vi "加速度信号处理.vi"(0 "输入信号":dbl[](graph), 1 "n":i32=2) -> (6 "滤波":dbl[](graph), 7 "重心频率FC":dbl, 8 "幅度谱":dbl[](graph), 9 "均方频率MSF":dbl, 10 "相位谱":dbl[](graph), 11 "去均值":dbl[](graph), 12 "功率谱":dbl[](graph), 13 "频率方差VF":dbl, 14 "均方根值":dbl format="%f", 15 "峰值指标":dbl format="%0.2p", 16 "峭度指标":dbl format="%0.2p", 17 "波形指标":dbl format="%0.2p", 18 "脉冲指标":dbl format="%0.2p", 19 "裕度指标":dbl format="%0.2p")   [LabVIEW 2014]
uses:
  <vilib>/Analysis/3filter.llb/Filter Passband Type.ctl
  <vilib>/Analysis/2dsp.llb/Power Spectrum (DBL).vi
  <vilib>/Analysis/3filter.llb/Butterworth Filter (DBL).vi
  <vilib>/measure/madcrms.llb/Basic Averaged DC-RMS for 1 Chan.vi
  <vilib>/Analysis/NI_AALBase.lvlib
  <vilib>/measure/NI_MAPro.lvlib
  <vilib>/Analysis/NI_AALPro.lvlib
panel:
  out "Power Spectrum":dbl[](array[numeric]) caption="功率谱"
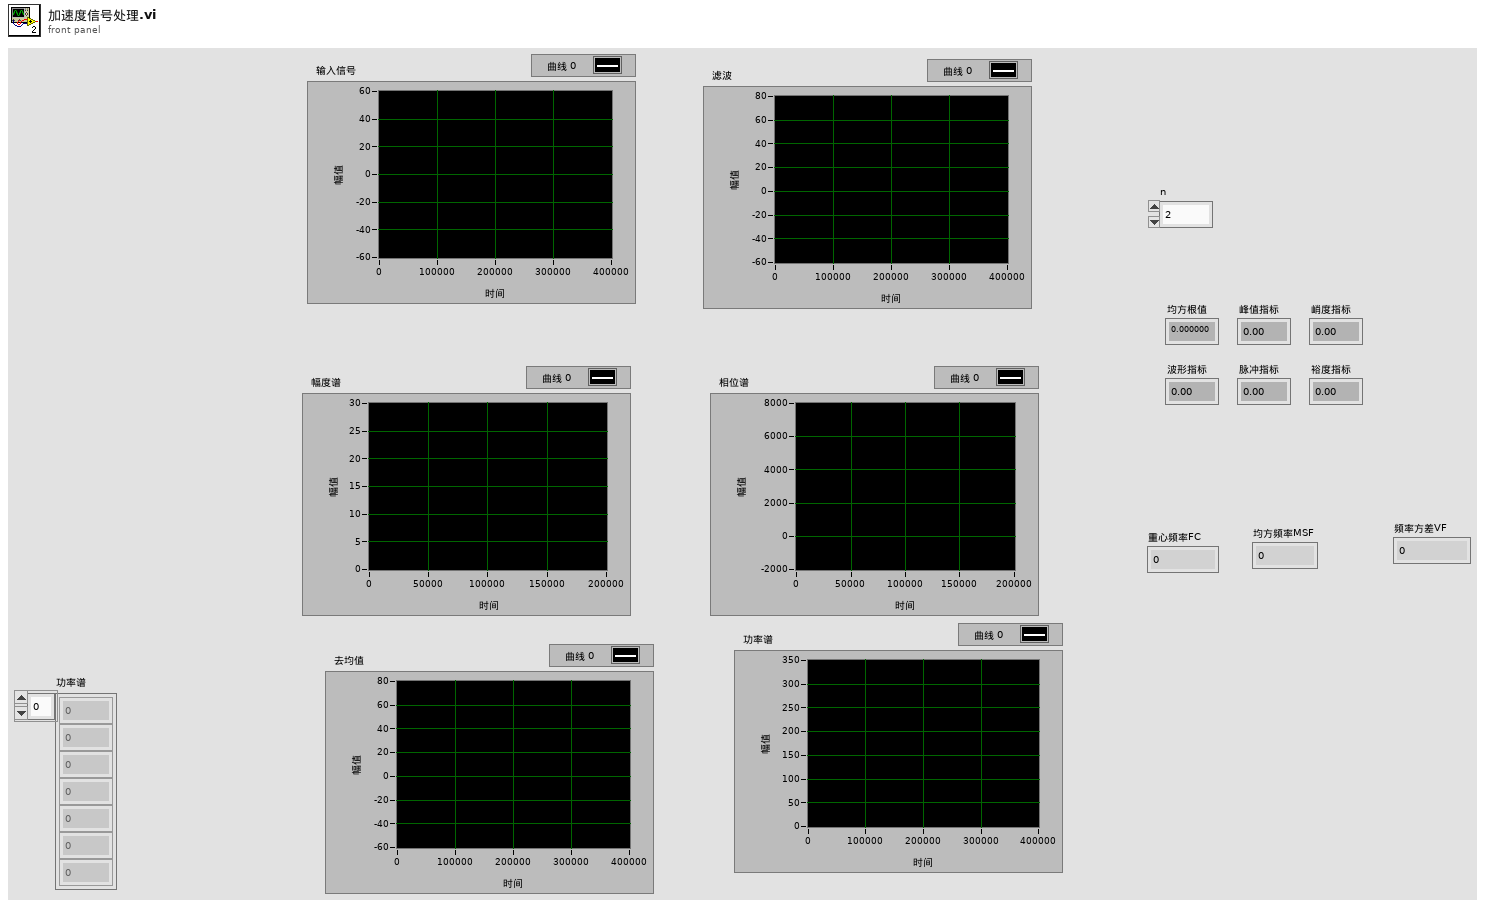
[diagram p1: front panel]
types:
  T1 = typedef "NI_AALBase.lvlib/Filter Passband Type.ctl" = enum32{"Lowpass", "Highpass", "Bandpass", "Bandstop"}
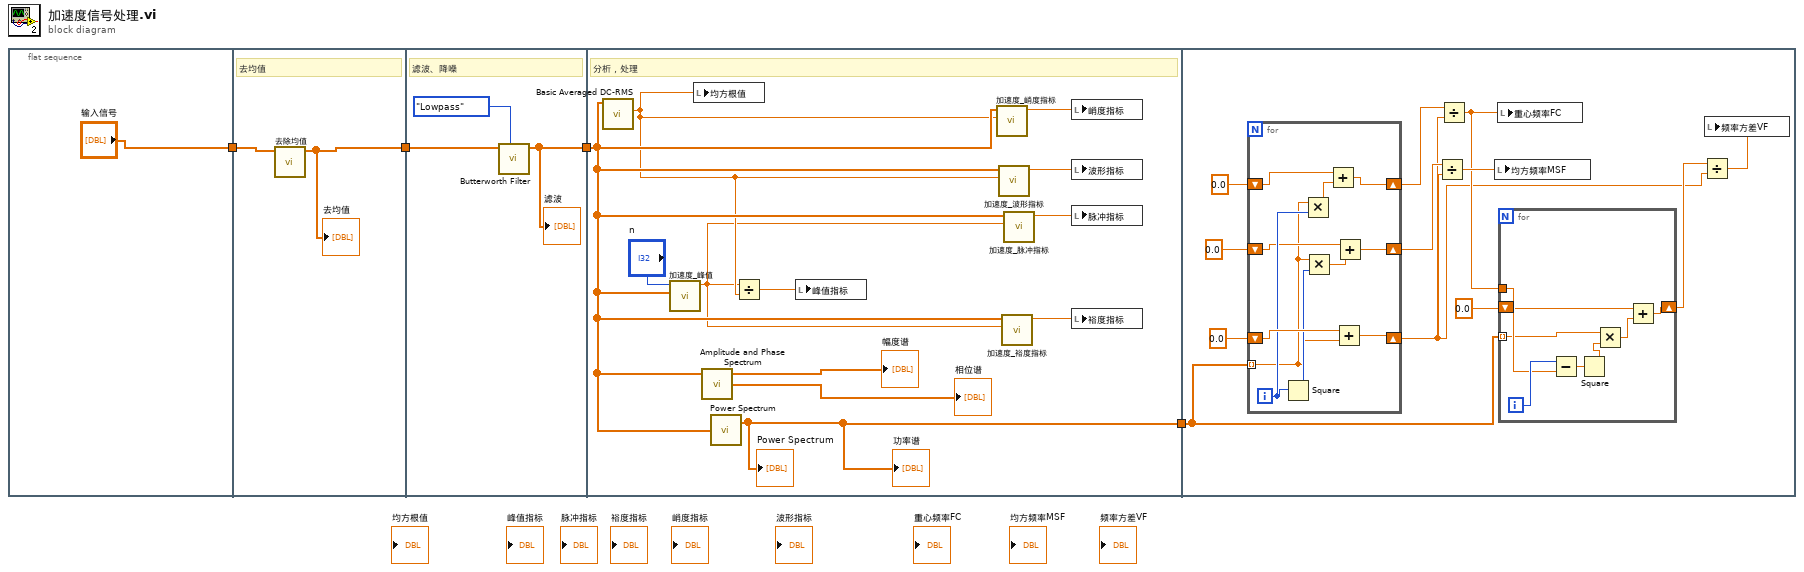
[diagram p0: block diagram]
diagram:
  n1 = flat-sequence {
    tunnel: ["输入信号"] -> w4
    tunnel: w4 -> [w7]
    tunnel: [w6] -> w3
    tunnel: w3 -> [w10]
    tunnel: [w8] -> w2
    tunnel: w2 -> [w16]
    tunnel: [w11] -> w1
    tunnel: w1 -> [w28]
    frame #0 {
    }
    frame #1 {
      # "去均值"
      n2 = call "去除均值.vi"("输入信号"=w7) -> ("去均值信号"=w6:dbl[])  [unwired: 10 in]
      "去均值" <- w6
    }
    frame #2 {
      # "滤波、降噪"
      n3 = call-poly <vilib>:"Butterworth Filter.vi"("filter type"=Filter_Passband_Type."Lowpass", "X"=w10) -> ("Filtered X"=w8:dbl[])  [unwired: 6 in, 1 out]
      "滤波" <- w8
    }
    frame #3 {
      # "分析，处理"
      n4 = call-poly <vilib>:"Basic Averaged DC-RMS.vi"("signal in"=w16) -> ("RMS value"=w14:dbl)  [unwired: 7 in, 3 out]
      n5 = call "加速度_峰值.vi"("信号X"=w16, "n"="n") -> ("峰值"=w12:dbl)  [unwired: 9 in]
      n6 = local write "均方根值"(w14) -> ()
      n7 = call <vilib>:"Amplitude and Phase Spectrum.vi"("Signal (V)"=w16) -> ("Amp Spectrum Phase (radians)"=→"相位谱":dbl[], "Amp Spectrum Mag (Vrms)"=→"幅度谱":dbl[])  [unwired: 2 in, 1 out]
      n8 = call-poly <vilib>:"Power Spectrum.vi"("X"=w16) -> ("Power Spectrum"=w11:dbl[])  [unwired: 1 out]
      "Power Spectrum" <- w11
      "功率谱" <- w11
      n9 = Divide(x=w12, y=w14) -> (x/y=w13:dbl)
      n10 = local write "峰值指标"(w13) -> ()
      n11 = call "加速度_峭度指标.vi"("均方根值"=w14, "信号X"=w16) -> ("峭度指标"=w22:dbl)  [unwired: 9 in]
      n12 = call "加速度_波形指标.vi"("均方根值"=w14, "信号X"=w16) -> ("波形指标"=w21:dbl)  [unwired: 9 in]
      n13 = call "加速度_裕度指标.vi"("峰值"=w12, "信号X"=w16) -> ("裕度指标"=w20:dbl)  [unwired: 9 in]
      n14 = call "加速度_脉冲指标.vi"("峰值"=w12, "信号X"=w16) -> ("脉冲指标"=w19:dbl)  [unwired: 9 in]
      n15 = local write "峭度指标"(w22) -> ()
      n16 = local write "波形指标"(w21) -> ()
      n17 = local write "脉冲指标"(w19) -> ()
      n18 = local write "裕度指标"(w20) -> ()
    }
    frame #4 {
      n19 = for {
        tunnel: w28 -> [w44] mode=indexing
        shift-right: [w52] -> w32
        shift-left: 0.0 -> [w53]
        shift-right: [w49] -> w24
        shift-left: 0.0 -> [w50]
        shift-right: [w47] -> w30
        shift-left: 0.0 -> [w46]
        i -> [w48]
        n20 = Square(x=w48) -> (x^2=w45:i32)
        n21 = Multiply(x=w44, y=w48) -> (x*y=w51:dbl)
        n22 = Multiply(x=w44, y=w45) -> (x*y=w43:dbl)
        n23 = Add(x=w53, y=w51) -> (x+y=w52:dbl)
        n24 = Add(x=w50, y=w44) -> (x+y=w49:dbl)
        n25 = Add(x=w46, y=w43) -> (x+y=w47:dbl)
      }
      n26 = Divide(x=w30, y=w24) -> (x/y=w29:dbl)
      n27 = Divide(x=w32, y=w24) -> (x/y=w27:dbl)
      n28 = local write "均方频率MSF"(w29) -> ()
      n29 = local write "重心频率FC"(w27) -> ()
      n30 = for {
        tunnel: w28 -> [w38] mode=indexing
        tunnel: w27 -> [w41]
        shift-right: [w35] -> w25
        shift-left: 0.0 -> [w36]
        i -> [w42]
        n31 = Subtract(x=w42, y=w41) -> (x-y=w40:dbl)
        n32 = Square(x=w40) -> (x^2=w39:dbl)
        n33 = Multiply(x=w38, y=w39) -> (x*y=w37:dbl)
        n34 = Add(x=w36, y=w37) -> (x+y=w35:dbl)
      }
      n35 = Divide(x=w25, y=w24) -> (x/y=w23:dbl)
      n36 = local write "频率方差VF"(w23) -> ()
    }
  }
